vi "Binning.vi"(0 "Notifier Name":string, 7 "Binning":u8, 11 "Error In":errorcluster) -> (4 "Notifier Name DUP":string, 15 "Error Out":errorcluster)   [LabVIEW 2020]
uses:
  Hardware Configuration/Hardware Configuration Controls/Company.ctl
  IDS/IDS Controls/IDS Actions.ctl
  IDS/IDS Controls/IDS Parameters.ctl
  IDS/IDS Controls/IDS Parameter List.ctl
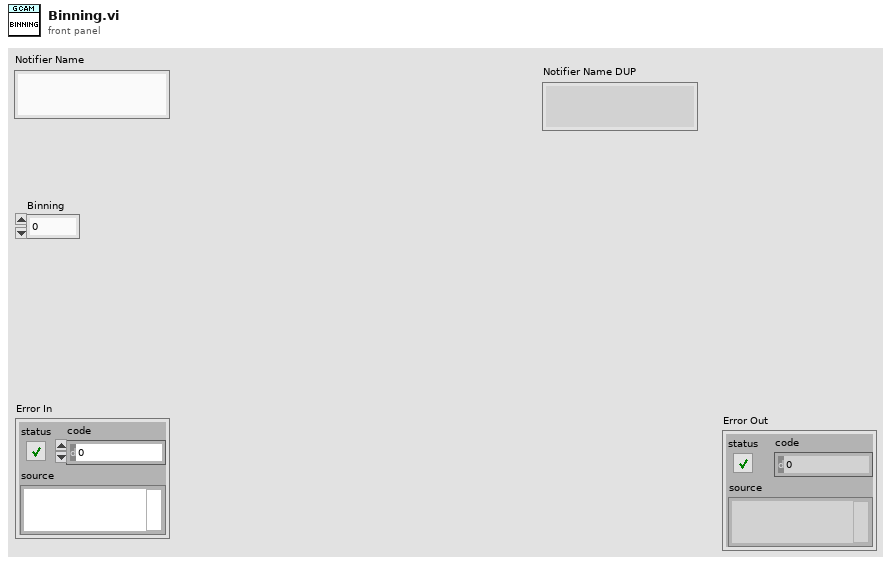
[diagram p1: front panel]
types:
  T1 = typedef "Company.ctl" = enum16{"AA Opto Electronic", "ASI", "Coherent", "Creset Optics", "CVI", "DAQmx", "Hamamatsu", "IDS", "Mad City Labs", "Marzhauser", "Measurement Computing", "MPB Com", "Olympus", "Photometrics", "PI", "Prior", "Thorlabs"}
  T2 = typedef "IDS Parameter List.ctl" = enum16{"Exposure Time (s)", "Binning"}
  T3 = typedef "IDS Parameters.ctl" = cluster{"Parameter":T2, "Value":dbl}
  T4 = typedef "IDS Actions.ctl" = enum16{"Error Check", "Initialize", "Preview", "Record", "Abort", "Record Settings", "Set Parameter", "Get Parameter", "Set ROI", "Get ROI", "Status", "Quit"}
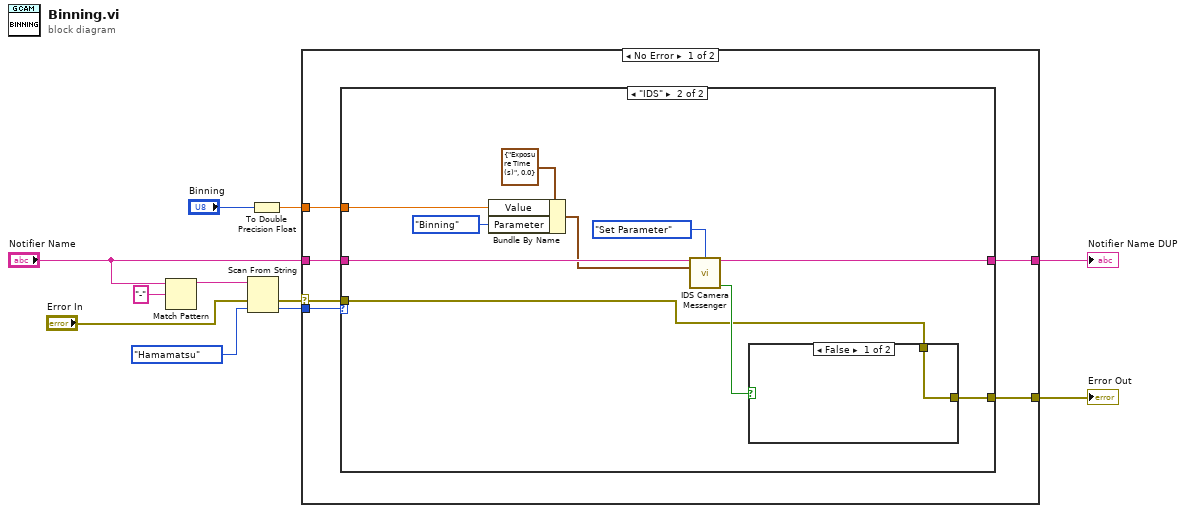
[diagram p0: block diagram]
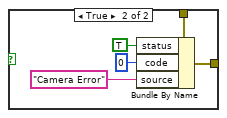
[diagram p3: hidden frame]
diagram:
  n1 = Match Pattern(string="Notifier Name", regular expression="-") -> (before substring=w9:string)  [unwired: 1 in, 3 out]
  n2 = Scan From String(input string=w9, error in="Error In", default 1=Company."Hamamatsu" ("Company")) -> (error out=w5:errorcluster, output 1=w8:T1)  [unwired: 2 in, 2 out]
  n3 = To Double Precision Float(number="Binning") -> (double precision float=w1:dbl)
  n4 = case shown="No Error" w5 {
    selector: w5 -> [w15 w36]
    tunnel: w8 -> [w17 _]
    tunnel: "Notifier Name" -> [w16 w37]
    tunnel: [w14 w37] -> w4
    tunnel: [w13 w36] -> w3
    tunnel: w1 -> [w12 _]
    frame No Error {
      n5 = case shown="\"IDS\"" w17 {
        tunnel: w16 -> [w19 w29]
        tunnel: w15 -> [w18 w25]
        tunnel: [w19 w28] -> w14
        tunnel: [w18 w24] -> w13
        tunnel: w12 -> [_ w22]
        frame Default {
        }
        frame "IDS" {
          n6 = Bundle By Name(cluster=T3 {"Parameter"=enum."Exposure Time (s)", "Value"=0.0} ("IDS Parameter"), "Value"=w22, "Parameter"=IDS_Parameter_List."Binning") -> (w20:T3)
          n7 = call "IDS Camera Messenger.vi"("Notifier Name"=w29, "IDS Actions"=IDS_Actions."Set Parameter", "IDS Parameter"=w20) -> ("Notifier Name (Dup)"=w28:string, "Error?"=w26:bool)  [unwired: 7 in, 4 out]
          n8 = case shown="False" w26 {
            tunnel: w25 -> [w30 w35]
            tunnel: [w30 w34] -> w24
            frame False {
            }
            frame True {
              n9 = Bundle By Name(cluster=w35, "status"=TRUE, "code"=0, "source"="Camera Error") -> (w34:errorcluster)
            }
          }
        }
      }
    }
    frame Error {
    }
  }
  "Error Out" <- w3
  "Notifier Name DUP" <- w4
